vi "UART Execute Command.vi"(0 "UART Driver in":refnum<class "UART Driver.lvclass">, 1 "Port Number":u8, 5 "Tx Data":string, 7 "Rx byte count":u32, 11 "error in":errorcluster) -> (4 "UART Driver out":refnum<class "UART Driver.lvclass">, 6 "Receive Data":string, 15 "error out":errorcluster)   [LabVIEW 2012, in "UART_Host_Driver.lvlib" / "UART Driver.lvclass"]
doc: "Performs a write and read operation to the port.\n\nMust call UART Initialize.vi and UART Configure Port.vi, prior to calling UART Execute Command.v\n\nNote: Port Number 255 means to transmit to all of the ports configured in the UART Initialize.vi."
uses:
  UART Driver.lvclass
  UART Driver.lvclass/UART Driver.ctl
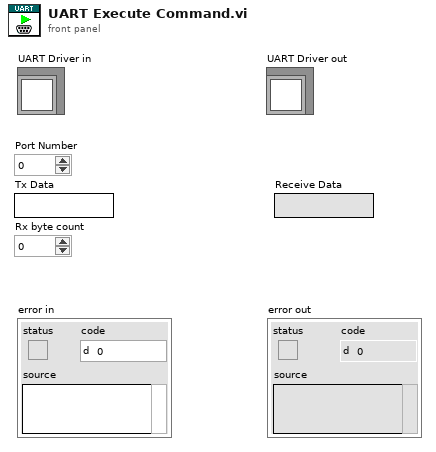
[diagram p1: front panel]
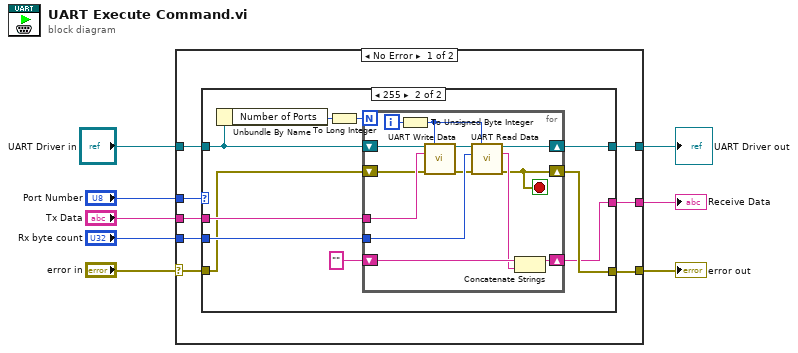
[diagram p0: block diagram]
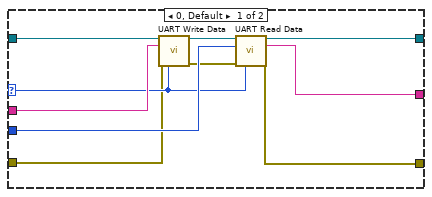
[diagram p2: hidden frame]
diagram:
  n1 = case shown="No Error" "error in" {
    selector: "error in" -> [w10 w50]
    tunnel: "Rx byte count" -> [w16 _]
    tunnel: [w15 _] -> w7
    tunnel: [w14 w51] -> w6
    tunnel: "Tx Data" -> [w13 _]
    tunnel: "UART Driver in" -> [w12 w51]
    tunnel: "Port Number" -> [w11 _]
    tunnel: [w9 w50] -> w1
    frame No Error {
      n2 = case shown="255" w11 {
        selector: w11 -> [w19 _]
        tunnel: w16 -> [w26 w36]
        tunnel: [w25 w27] -> w15
        tunnel: [w24 w35] -> w14
        tunnel: w13 -> [w21 w34]
        tunnel: w12 -> [w20 w31]
        tunnel: w10 -> [w18 w33]
        tunnel: [w17 w32] -> w9
        frame 0, Default {
          n3 = call-dynamic "UART Write Data.vi"("UART Driver in"=w20, "Port Number"=w19, "Tx Data"=w21, "error in"=w18) -> ("UART Driver out"=w22:refnum<class "UART Driver.lvclass">, "error out"=w23:errorcluster)  [unwired: 10 in]
          n4 = call-dynamic "UART Read Data.vi"("UART Driver in"=w22, "Port Number"=w19, "Rx byte count"=w26, "error in"=w23) -> ("UART Driver out"=w24:refnum<class "UART Driver.lvclass">, "Receive Data"=w25:string, "error out"=w17:errorcluster)  [unwired: 9 in]
        }
        frame 255 {
          n5 = Unbundle By Name(w31) -> ("Number of Ports"=w30:u8)
          n6 = To Long Integer(number=w30) -> (32bit integer=w29:i32)
          n7 = for {
            N: w29 -> [_]
            tunnel: w36 -> [w49]
            tunnel: w34 -> [w45]
            shift-right: [w39] -> w32
            shift-left: w33 -> [w44]
            shift-right: [w48] -> w35
            shift-left: w31 -> [w43]
            shift-right: [w41] -> w27
            shift-left: "" -> [w42]
            i -> [w38]
            stop <- w39 stop-if-true
            n8 = To Unsigned Byte Integer(number=w38) -> (unsigned 8bit integer=w37:u8)
            n9 = call-dynamic "UART Write Data.vi"("UART Driver in"=w43, "Port Number"=w37, "Tx Data"=w45, "error in"=w44) -> ("UART Driver out"=w46:refnum<class "UART Driver.lvclass">, "error out"=w47:errorcluster)  [unwired: 10 in]
            n10 = call-dynamic "UART Read Data.vi"("UART Driver in"=w46, "Port Number"=w37, "Rx byte count"=w49, "error in"=w47) -> ("UART Driver out"=w48:refnum<class "UART Driver.lvclass">, "Receive Data"=w40:string, "error out"=w39:errorcluster)  [unwired: 9 in]
            n11 = Concatenate Strings(w42, w40) -> (w41:string)
          }
        }
      }
    }
    frame Error {
    }
  }
  "Receive Data" <- w7
  "error out" <- w1
  "UART Driver out" <- w6
